vi "Y_AxisMoveTo.vi"(3 "Position":u32=100) -> ()   [LabVIEW 2020]
uses:
  C:/Program Files/National Instruments/LabVIEW 2020/examples/Instrument IO/Serial/support/Serial - Settings.ctl
  <vilib>/Instr/_visa.llb/VISA Configure Serial Port (Instr).vi
panel:
  in  "Serial Com Port":refnum<visa-resource-name>="COM3"
  in  "Serial Settings":T1={"baud rate"=57600, "data bits"=8, "parity"=enum."None", "stop bits"=10, "flow control"=0} {"flow control" items=["None"=0, "XON/XOFF"=1, "RTS/CTS"=2, "DTR/DSR"=4]; "stop bits" items=["1.0"=10, "1.5"=15, "2.0"=20]; "data bits" min=5 max=8 step=1; "baud rate" items=["75"=75, "110"=110, "134"=134, "150"=150, "300"=300, "600"=600, "1200"=1200, "1800"=1800, "2400"=2400, "4800"=4800, "7200"=7200, "9600"=9600, "14400"=14400, "19200"=19200, "28800"=28800, "38400"=38400, "56000"=56000, "57600"=57600, "115200"=115200, "128000"=128000, "230400"=230400]}
  out "Finished":bool
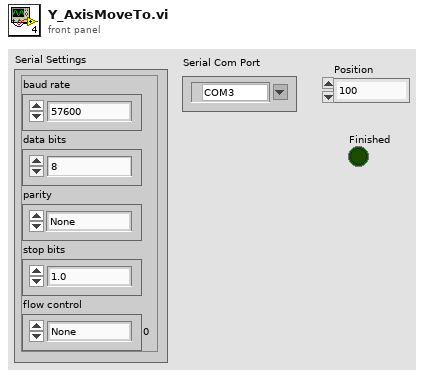
[diagram p1: front panel]
types:
  T1 = typedef "Serial - Settings.ctl" = cluster{"baud rate":u32, "data bits":u16, "parity":enum16{"None", "Odd", "Even", "Mark", "Space"}, "stop bits":u16, "flow control":u16}
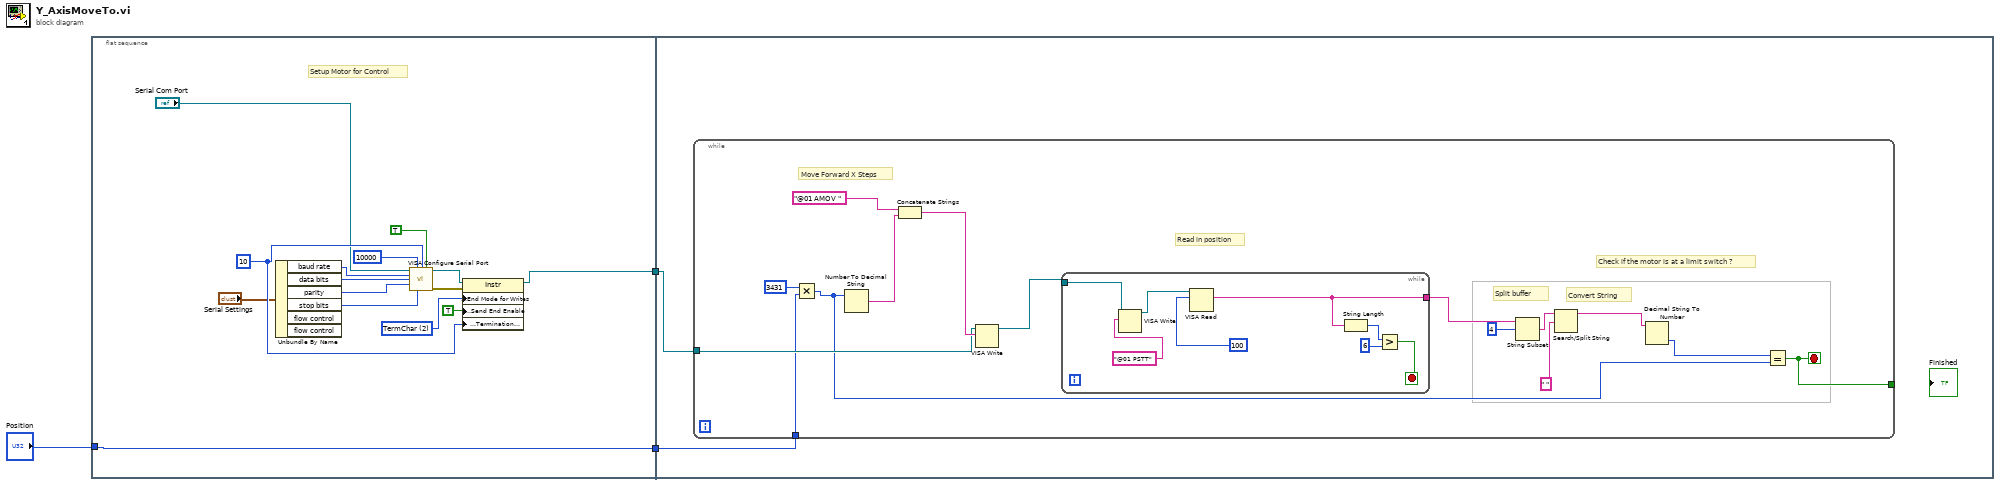
[diagram p0: block diagram]
diagram:
  n1 = flat-sequence {
    tunnel: [w5] -> w3
    tunnel: "Position" -> [w4]
    tunnel: [w4] -> w1
    tunnel: w3 -> [w20]
    tunnel: w1 -> [w19]
    frame #0 {
      w9 = u8 10 ("Termination Character")
      w13 = u16 2 items=["None", "LastBit", "TermChar", "Break"] ("Serial Settings:Serial End Mode for Writes")
      # "Setup Motor for Control"
      n2 = Unbundle By Name("Serial Settings") -> ("baud rate"=w15:u32, "data bits"=w16:u16, "parity"=w17:enum16{"None", "Odd", "Even", "Mark", "Space"}, "stop bits"=w18:u16)  [unwired: 2 out]
      n3 = call-poly "VISA Configure Serial Port"("VISA resource name"="Serial Com Port", "timeout (10sec)"=u32 10000, "termination char\n(0xA = '\\n' = LF)"=w9, "Enable Termination\nChar (T)"=TRUE ("End Read on Termination Character?"), "baud rate (9600)"=w15, "data bits (8)"=w16, "parity (0:none)"=w17, "stop bits (10: 1 bit)"=w18) -> ("VISA resource name out"=w6:refnum<visa-resource-name>, "error out"=w14:errorcluster)  [unwired: 2 in, 4 out]
      n4 = property class="Instr"(reference=w6, error in=w14, "Serial Settings:End Mode for Writes"=w13, "Message Based Settings:Send End Enable"=TRUE, "Message Based Settings:Termination Character"=w9) -> (reference out=w5:refnum<visa-resource-name>)  [unwired: 1 out]
    }
    frame #1 {
      n5 = while {
        tunnel: [w35] -> _
        tunnel: w20 -> [w24]
        tunnel: w19 -> [w23]
        stop <- w35 stop-if-true
        # "Move Forward X Steps"
        # "Check if the motor is at a limit switch ?"
        # "Read in position"
        # "Convert String"
        # "Split buffer"
        n6 = Multiply(x=u32 3431, y=w23) -> (x*y=w21:u32)
        n7 = Number To Decimal String(number=w21) -> (decimal integer string=w28:string)  [unwired: 1 in]
        n8 = Concatenate Strings("@01 AMOV " ("Command 2"), w28) -> (w27:string)
        n9 = VISA Write(VISA resource name=w24, write buffer=w27) -> (VISA resource name out=w25:refnum<visa-resource-name>)  [unwired: 1 in, 2 out]
        n10 = while {
          tunnel: [w40] -> w32
          tunnel: w25 -> [w36]
          stop <- w39 stop-if-true
          n11 = VISA Write(VISA resource name=w36, write buffer="@01 PSTT" ("Command 2")) -> (VISA resource name out=w38:refnum<visa-resource-name>)  [unwired: 1 in, 2 out]
          n12 = VISA Read(VISA resource name=w38, byte count=u32 100 ("Read Word Length Count?")) -> (read buffer=w40:string)  [unwired: 1 in, 3 out]
          n13 = String Length(string=w40) -> (length=w42:i32)
          n14 = Greater?(x=w42, y=6) -> (0:w39:bool)
        }
        n15 = String Subset(string=w32, offset (0)=4) -> (substring=w30:string)  [unwired: 1 in]
        n16 = Search/Split String(string=w30, search string/char (-)=" ") -> (substring before match=w29:string)  [unwired: 1 in, 2 out]
        n17 = Decimal String To Number(string=w29) -> (number=w34:i32)  [unwired: 2 in, 1 out]
        n18 = Equal?(x=w34, y=w21) -> (x = y?=w35:bool)
      }
    }
  }
